vi "Main.vi"() -> ()   [LabVIEW 2014, in "1. Constructing and Using a Widget.lvlib"]
doc: "Widgets are versatile building blocks for GUIs. Each widget can act as a standalone window (just like a VI's front panel), or it can be embedded into a larger widget (just like a control/ indicator) to create a complex GUI.\n\nThis example simply contains one standalone widget. Later examples will show you how to compose a GUI using multiple widgets.\n\n\nCopyright (c) 2019 Sze Howe Koh.\nThis code is licensed under the MIT license."
uses:
  1. Constructing and Using a Widget.lvlib
  <vilib>/addons/LQ/LQ Core/QSize.ctl
  <vilib>/addons/LQ/Qt Widgets/QWidget/resize.vi
  <vilib>/addons/LQ/Qt Widgets/QWidget/setVisible.vi
  <vilib>/addons/LQ/LQ Core/LQCoreEngine/LQCoreEngine.lvclass
  <vilib>/addons/LQ/Qt Widgets/QLCDNumber/QLCDNumber.lvclass
panel:
  in  "Stop Button":bool
  # "Prerequisite knowledge/experience\n- Basic LabVIEW programming\n\n\nDescription\nWidgets are versatile building blocks for GUIs. Each widget can act as a\nstandalone window (just like a VI's front panel), or it can be embedded\ninto a larger widget (just like a control/ indicator) to create a complex GUI.\n\nThis example simply contains one standalone widget. Later examples will\nshow you how to compose a GUI using multiple widgets.\n\n\nInstructions\n1. Run this VI and watch the LCD widget.\n2. Use your mouse to resize the widget.\n3. Click \"Stop\"."
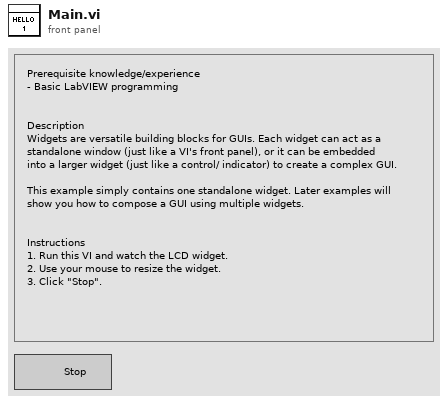
[diagram p1: front panel]
types:
  T1 = typedef "QSize.ctl" = cluster{"width":i32, "height":i32}
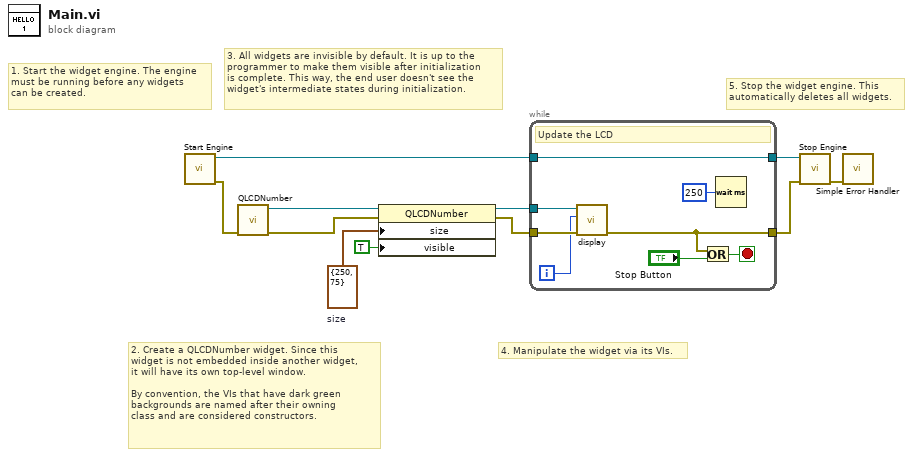
[diagram p0: block diagram]
diagram:
  w5 = T1 {"width"=250, "height"=75}  # size
  # "4. Manipulate the widget via its VIs."
  # "3. All widgets are invisible by default. It is up to the\nprogrammer to make them visible after initialization\nis complete. This way, the end user doesn't see the\nwidget's intermediate states during initialization."
  # "2. Create a QLCDNumber widget. Since this\nwidget is not embedded inside another widget,\nit will have its own top-level window.\n\nBy convention, the VIs that have dark green\nbackgrounds are named after their owning\nclass and are considered constructors."
  # "5. Stop the widget engine. This\nautomatically deletes all widgets."
  # "1. Start the widget engine. The engine\nmust be running before any widgets\ncan be created."
  n1 = call <vilib>:"Start Engine.vi"() -> ("Error Out"=w8:errorcluster, "New Engine"=w10:refnum<class "LQCoreEngine.lvclass">)  [unwired: 10 in]
  n2 = call <vilib>:"QLCDNumber.vi"("Error In"=w8) -> ("Error Out"=w11:errorcluster, "New QLCDNumber"=w2:refnum<class "QLCDNumber.lvclass">)  [unwired: 9 in]
  n3 = property class="QLCDNumber"(reference=w2, error in=w11, "size"=w5, "visible"=TRUE) -> (reference out=w1:refnum<class "QLCDNumber.lvclass">, error out=w7:errorcluster)
  n4 = while {
    tunnel: w7 -> [w14]
    tunnel: [w13] -> w3
    tunnel: w1 -> [w15]
    tunnel: w10 -> [w19]
    tunnel: [w19] -> w9
    i -> [w12]
    stop <- w17 stop-if-true
    # "Update the LCD"
    n5 = call <vilib>:"display.vi"("Error In"=w14, "num"=w12, "QLCDNumber In"=w15) -> ("Error Out"=w13:errorcluster)  [unwired: 7 in, 1 out]
    n6 = Or(x=w13, y="Stop Button") -> (x .or. y?=w17:bool)
    n7 = Wait (ms)(milliseconds to wait=u32 250) -> ()  [unwired: 1 out]
  }
  n8 = call <vilib>:"Stop Engine.vi"("Error In"=w3, "LQCoreEngine"=w9) -> ("Error Out"=w6:errorcluster)  [unwired: 9 in]
  n9 = call <vilib>:"Simple Error Handler.vi"("error in (no error)"=w6) -> ()  [unwired: 4 in, 5 out]
